vi "CreateVerifyVersionMessage.vi"(8 "error in (no error)":errorcluster, 9 "reply to":string, 10 "device name":string, 11 "prov version info":T1) -> (0 "error out":errorcluster, 3 "message":T2)   [LabVIEW 2017, in "ServerComm.lvlib"]
uses:
  <vilib>/addons/InsightCM/Devices/Shared/Common/ServerComm/ServerComm.lvlib
  <vilib>/addons/InsightCM/MessageBus/Base/controls/Message.ctl
  <vilib>/addons/InsightCM/MessageBus/Base/controls/MessageHeader.ctl
  <vilib>/addons/InsightCM/MessageBus/Base/controls/KeyValuePair.ctl
  <vilib>/addons/InsightCM/Devices/Shared/Common/ServerComm/controls/ProvisioningVersionInfo.ctl
  <vilib>/addons/InsightCM/MessageBus/MessageLibrary/Provisioning/controls/ProvisioningVerifyVersionsRequestBody.ctl
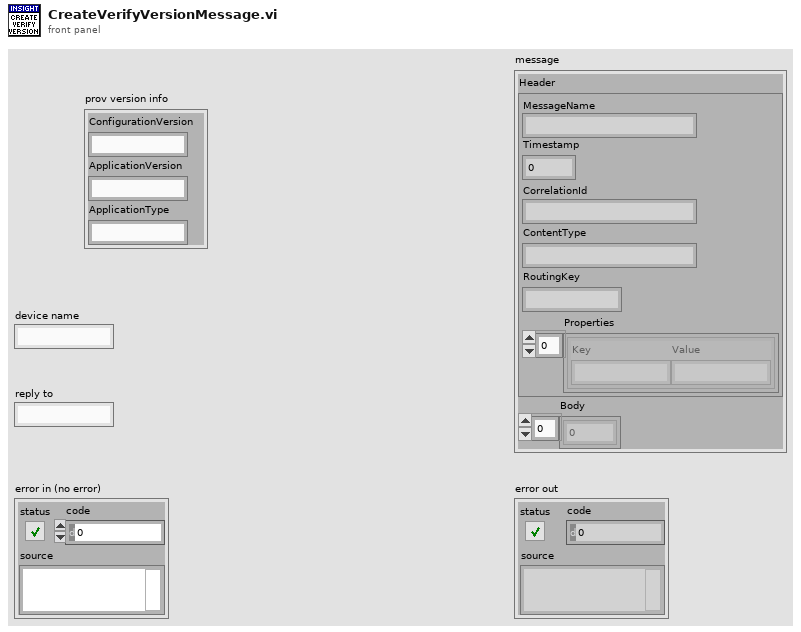
[diagram p1: front panel]
types:
  T1 = typedef "ServerComm.lvlib/ProvisioningVersionInfo.ctl" = cluster{"ConfigurationVersion":string, "ApplicationVersion":string, "ApplicationType":string}
  T2 = typedef "Message.ctl" = cluster{"Header":T3, "Body":u8[]}
  T3 = typedef "MessageHeader.ctl" = cluster{"MessageName":string, "Timestamp":i64, "CorrelationId":string, "ContentType":string, "RoutingKey":string, "Properties":T4[]}
  T4 = typedef "KeyValuePair.ctl" = cluster{"Key":string, "Value":string}
  T5 = typedef "ProvisioningVerifyVersionsRequestBody.ctl" = cluster{"DeviceName":string, "ApplicationType":string, "ApplicationVersion":string, "ConfigurationVersion":string}
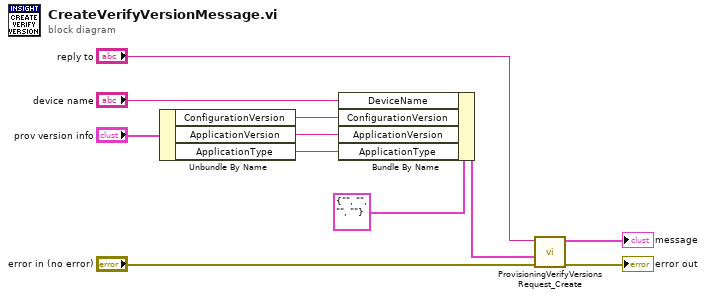
[diagram p0: block diagram]
diagram:
  n1 = Unbundle By Name("prov version info") -> ("ConfigurationVersion"=w10:string, "ApplicationVersion"=w9:string, "ApplicationType"=w8:string)
  n2 = Bundle By Name(cluster=T5 {"DeviceName"="", "ApplicationType"="", "ApplicationVersion"="", "ConfigurationVersion"=""} ("ProvisioningVerifyVersionsRequest"), "DeviceName"="device name", "ConfigurationVersion"=w10, "ApplicationVersion"=w9, "ApplicationType"=w8) -> (w7:T5)
  n3 = call <vilib>:"ProvisioningVerifyVersionsRequest_Create.vi"("error in (no error)"="error in (no error)", "ProvisioningVerifyVersionsRequest"=w7, "ReplyTo"="reply to") -> ("error out"=→"error out":errorcluster, "Message"=→"message":T2)  [unwired: 7 in]
